vi "subRegist_UserInfo.vi"(10 "user name":string, 11 "log path":path) -> ()   [LabVIEW 2015]
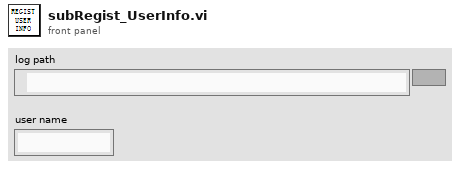
[diagram p1: front panel]
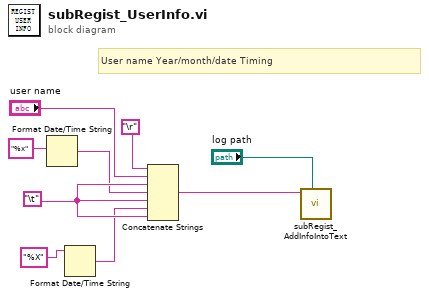
[diagram p0: block diagram]
diagram:
  w7 = "\t"
  # "User name Year/month/date Timing"
  n1 = Format Date/Time String(time format string (%c)="%x") -> (date/time string=w4:string)  [unwired: 2 in]
  n2 = Format Date/Time String(time format string (%c)="%X") -> (date/time string=w6:string)  [unwired: 2 in]
  n3 = Concatenate Strings("\r", "user name", w7, w4, w7, w6, w7) -> (w1:string)
  n4 = call "subRegist_AddInfoIntoText.vi"("log path"="log path", "info to be added"=w1) -> ()  [unwired: 10 in]
